vi "MotorNavigation.vi"() -> ()   [LabVIEW 2022 SP3]
panel:
  in  "Zero":bool
  in  "TZ [mm]":dbl format="%.3f"
  in  "TY [mm]":dbl format="%.3f"
  in  "TX [mm]":dbl format="%.3f"
  in  "SZ":u16(ring)=4000 items=["4000 ustep/s"=4000, "2000 ustep/s"=2000, "1000 ustep/s"=1000]
  in  "SY":u16(ring)=4000 items=["4000 ustep/s"=4000, "2000 ustep/s"=2000, "1000 ustep/s"=1000]
  in  "SX":u16(ring)=4000 items=["6000 ustep/s"=6000, "4000 ustep/s"=4000, "2000 ustep/s"=2000, "1000 ustep/s"=1000]
  out "Z [mm]":dbl format="%.3f"
  out "Y [mm]":dbl format="%.3f"
  out "X [mm]":dbl format="%.3f"
  in  "ustepZ":u16(ring)=4 items=["full"=1, "1/2"=2, "1/4"=4, "1/8"=8, "1/16"=16]
  in  "ustepY":u16(ring)=4 items=["full"=1, "1/2"=2, "1/4"=4, "1/8"=8, "1/16"=16]
  in  "ustepX":u16(ring)=4 items=["full"=1, "1/2"=2, "1/4"=4, "1/8"=8, "1/16"=16]
  in  "Abort":bool
  out "Moving":bool
  in  "Motor VISA":refnum<visa-resource-name>="COM4"
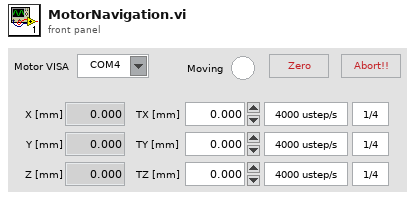
[diagram p1: front panel]
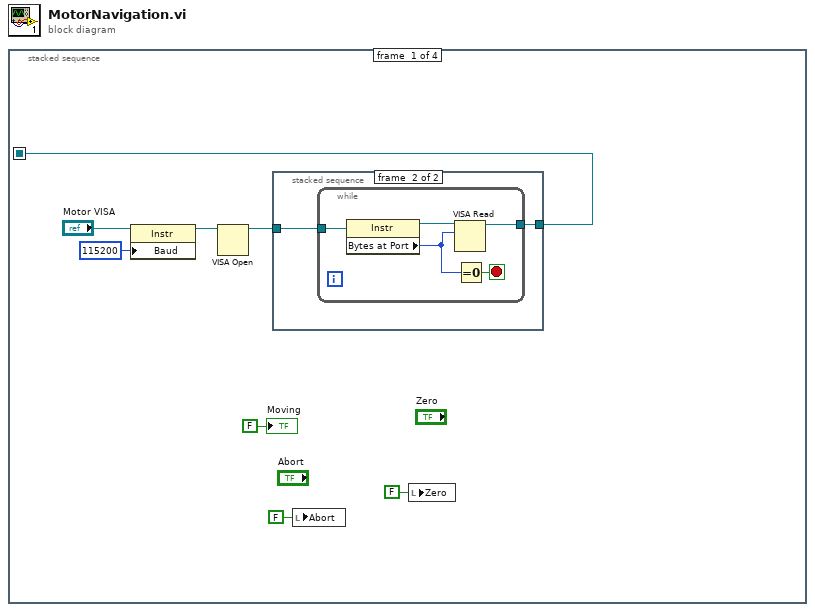
[diagram p0: block diagram]
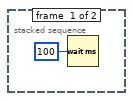
[diagram p2: hidden frame]
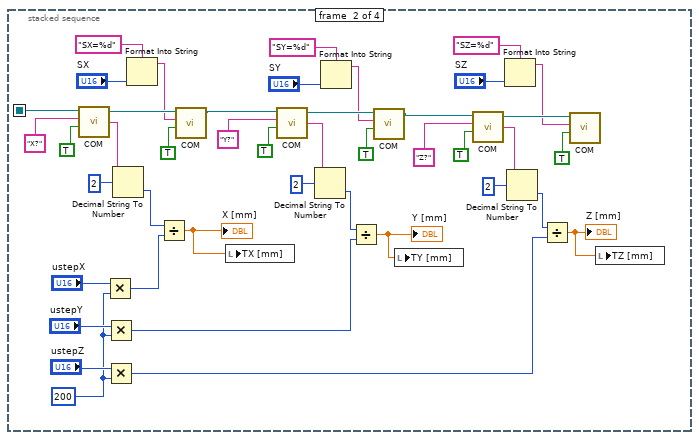
[diagram p3: hidden frame]
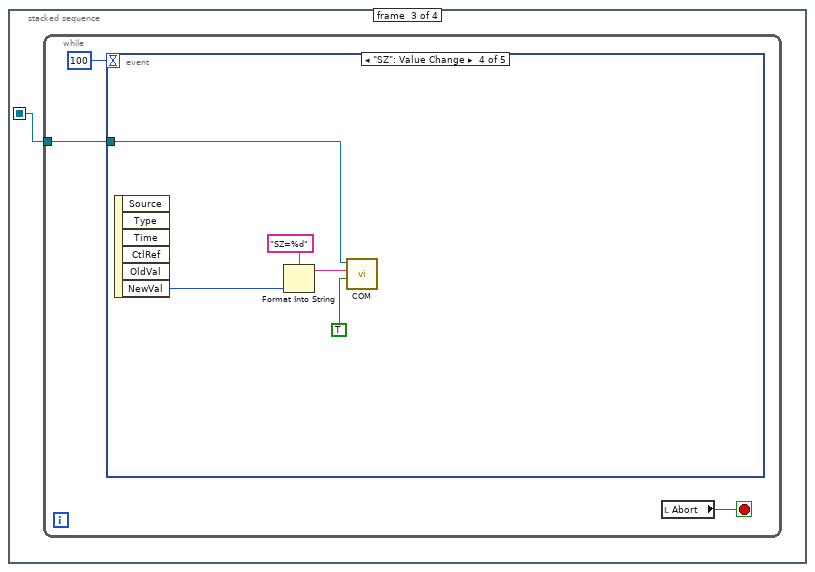
[diagram p4: hidden frame]
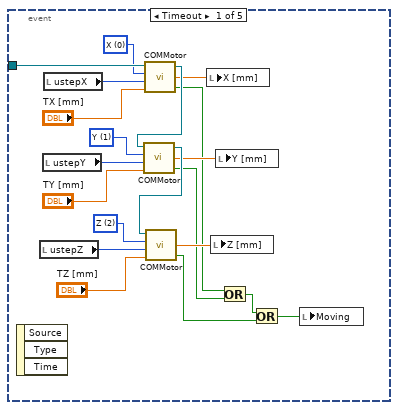
[diagram p5: hidden frame]
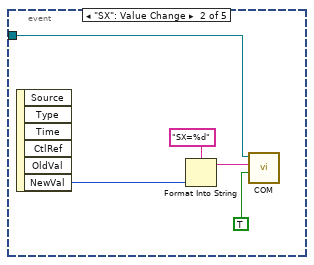
[diagram p6: hidden frame]
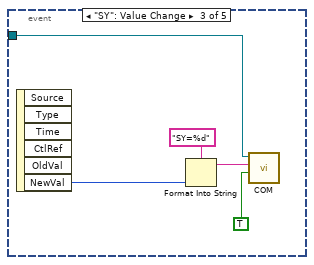
[diagram p7: hidden frame]
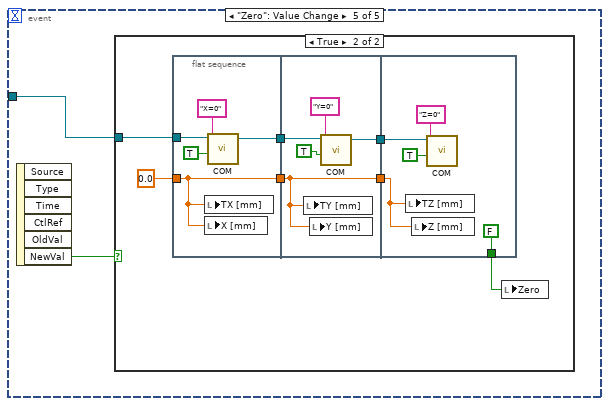
[diagram p8: hidden frame]
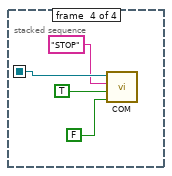
[diagram p10: hidden frame]
diagram:
  n1 = stacked-sequence {
    seq-local: [w4 _ _ _] -> [_ w59 w60 w126]
    frame #0 {
      n2 = property class="Instr"(reference="Motor VISA", "Baud"=u32 115200 ("Serial Settings:Baud Rate")) -> (reference out=w6:refnum<visa-resource-name>)  [unwired: 1 in, 1 out]
      n3 = VISA Open(VISA resource name=w6) -> (VISA resource name=w5:refnum<visa-resource-name>)  [unwired: 4 in, 1 out]
      n4 = stacked-sequence {
        tunnel: w5 -> [_ w11]
        tunnel: [_ w10] -> w4
        frame #0 {
          n5 = Wait (ms)(milliseconds to wait=u32 100) -> ()  [unwired: 1 out]
        }
        frame #1 {
          n6 = while {
            tunnel: w11 -> [w16]
            tunnel: [w12] -> w10
            stop <- w13 stop-if-true
            n7 = property class="Instr"(reference=w16) -> (reference out=w15:refnum<visa-resource-name>, "Bytes at Port"=w14:u32)  [unwired: 1 in, 1 out]
            n8 = VISA Read(VISA resource name=w15, byte count=w14) -> (VISA resource name out=w12:refnum<visa-resource-name>)  [unwired: 1 in, 3 out]
            n9 = Equal To 0?(x=w14) -> (x = 0?=w13:bool)
          }
        }
      }
      n10 = local write "Abort"(FALSE ("Abort")) -> ()
      n11 = local write "Zero"(FALSE ("Zero")) -> ()
      "Moving" <- FALSE ("Moving")
    }
    frame #1 {
      w39 = 200
      n12 = call "COM.vi"("Write?"=TRUE, "command"="X?", "VISA in"=w59) -> ("reply"=w44:string, "VISA out"=w55:refnum<visa-resource-name>)  [unwired: 1 in, 1 out]
      n13 = Multiply(x="ustepX", y=w39) -> (x*y=w37:i32)
      n14 = Multiply(x="ustepY", y=w39) -> (x*y=w31:i32)
      n15 = Multiply(x="ustepZ", y=w39) -> (x*y=w29:i32)
      n16 = Decimal String To Number(string=w44, offset=2 ("offset (0)")) -> (number=w38:i32)  [unwired: 1 in, 1 out]
      n17 = Format Into String(format string="SX=%d" ("command"), "SX") -> (resulting string=w26:string)  [unwired: 2 in, 1 out]
      n18 = Divide(x=w38, y=w37) -> (x/y=w19:dbl)
      "X [mm]" <- w19
      n19 = call "COM.vi"("Write?"=TRUE, "command"=w26, "VISA in"=w55) -> ("VISA out"=w46:refnum<visa-resource-name>)  [unwired: 1 in, 2 out]
      n20 = local write "TX [mm]"(w19) -> ()
      n21 = call "COM.vi"("Write?"=TRUE, "command"="Y?", "VISA in"=w46) -> ("reply"=w34:string, "VISA out"=w51:refnum<visa-resource-name>)  [unwired: 1 in, 1 out]
      n22 = Decimal String To Number(string=w34, offset=2 ("offset (0)")) -> (number=w32:i32)  [unwired: 1 in, 1 out]
      n23 = Format Into String(format string="SY=%d" ("command"), "SY") -> (resulting string=w21:string)  [unwired: 2 in, 1 out]
      n24 = Divide(x=w32, y=w31) -> (x/y=w17:dbl)
      "Y [mm]" <- w17
      n25 = call "COM.vi"("Write?"=TRUE, "command"=w21, "VISA in"=w51) -> ("VISA out"=w45:refnum<visa-resource-name>)  [unwired: 1 in, 2 out]
      n26 = local write "TY [mm]"(w17) -> ()
      n27 = call "COM.vi"("Write?"=TRUE, "command"="Z?", "VISA in"=w45) -> ("reply"=w33:string, "VISA out"=w47:refnum<visa-resource-name>)  [unwired: 1 in, 1 out]
      n28 = Format Into String(format string="SZ=%d" ("command"), "SZ") -> (resulting string=w20:string)  [unwired: 2 in, 1 out]
      n29 = Decimal String To Number(string=w33, offset=2 ("offset (0)")) -> (number=w30:i32)  [unwired: 1 in, 1 out]
      n30 = Divide(x=w30, y=w29) -> (x/y=w18:dbl)
      "Z [mm]" <- w18
      n31 = call "COM.vi"("Write?"=TRUE, "command"=w20, "VISA in"=w47) -> ()  [unwired: 1 in, 3 out]
      n32 = local write "TZ [mm]"(w18) -> ()
    }
    frame #2 {
      n33 = while {
        tunnel: w60 -> [w62]
        stop <- w61 stop-if-true
        n34 = event shown="[3] \"SZ\": Value Change" {
          selector: _ -> [_ _ _ _ _]
          dyn-events: _ -> [_ _ _ _ _]
          timeout: 100 -> [_ _ _ _ _]
          tunnel: w62 -> [w80 w85 w90 w95 w99]
          event Timeout {
            w73 = u16 2 items=["X", "Y", "Z"] ("axis")
            w77 = u16 1 items=["X", "Y", "Z"] ("axis")
            w79 = u16 0 items=["X", "Y", "Z"] ("axis")
            n35 = event-data() -> ()  [unwired: 1 in, 3 out]
            n36 = local read "ustepZ"() -> (w74:u16)
            n37 = local read "ustepY"() -> (w76:u16)
            n38 = local read "ustepX"() -> (w78:u16)
            n39 = call "COMMotor.vi"("Target [mm]"="TX [mm]", "ustep"=w78, "axis"=w79, "VISA in"=w80) -> ("Moving"=w66:bool, "Position [mm]"=w81:dbl, "VISA out"=w83:refnum<visa-resource-name>)
            n40 = call "COMMotor.vi"("Target [mm]"="TY [mm]", "ustep"=w76, "axis"=w77, "VISA in"=w83) -> ("Moving"=w65:bool, "Position [mm]"=w69:dbl, "VISA out"=w75:refnum<visa-resource-name>)
            n41 = call "COMMotor.vi"("Target [mm]"="TZ [mm]", "ustep"=w74, "axis"=w73, "VISA in"=w75) -> ("Moving"=w64:bool, "Position [mm]"=w68:dbl)  [unwired: 1 out]
            n42 = local write "X [mm]"(w81) -> ()
            n43 = local write "Z [mm]"(w68) -> ()
            n44 = local write "Y [mm]"(w69) -> ()
            n45 = Or(x=w66, y=w65) -> (x .or. y?=w67:bool)
            n46 = Or(x=w67, y=w64) -> (x .or. y?=w82:bool)
            n47 = local write "Moving"(w82) -> ()
          }
          event "SX": Value Change {
            n48 = event-data() -> ("NewVal"=w87:u16)  [unwired: 1 in, 5 out]
            n49 = Format Into String(format string="SX=%d" ("command"), w87) -> (resulting string=w86:string)  [unwired: 2 in, 1 out]
            n50 = call "COM.vi"("Write?"=TRUE, "command"=w86, "VISA in"=w85) -> ()  [unwired: 1 in, 3 out]
          }
          event "SY": Value Change {
            n51 = event-data() -> ("NewVal"=w92:u16)  [unwired: 1 in, 5 out]
            n52 = Format Into String(format string="SY=%d" ("command"), w92) -> (resulting string=w91:string)  [unwired: 2 in, 1 out]
            n53 = call "COM.vi"("Write?"=TRUE, "command"=w91, "VISA in"=w90) -> ()  [unwired: 1 in, 3 out]
          }
          event "SZ": Value Change {
            n54 = event-data() -> ("NewVal"=w97:u16)  [unwired: 1 in, 5 out]
            n55 = Format Into String(format string="SZ=%d" ("command"), w97) -> (resulting string=w96:string)  [unwired: 2 in, 1 out]
            n56 = call "COM.vi"("Write?"=TRUE, "command"=w96, "VISA in"=w95) -> ()  [unwired: 1 in, 3 out]
          }
          event "Zero": Value Change {
            n57 = event-data() -> ("NewVal"=w100:bool)  [unwired: 1 in, 5 out]
            n58 = case shown="True" w100 {
              tunnel: w99 -> [_ w107]
              frame False {
              }
              frame True {
                n59 = flat-sequence {
                  tunnel: w107 -> [w112]
                  tunnel: 0.0 ("TX [mm]") -> [w110]
                  tunnel: [w110] -> w105
                  tunnel: [w108] -> w103
                  tunnel: w105 -> [w117]
                  tunnel: [w117] -> w104
                  tunnel: w103 -> [w114]
                  tunnel: [w113] -> w102
                  tunnel: w104 -> [w122]
                  tunnel: w102 -> [w119]
                  tunnel: [FALSE ("Zero")] -> w101
                  frame #0 {
                    n60 = local write "TX [mm]"(w110) -> ()
                    n61 = local write "X [mm]"(w110) -> ()
                    n62 = call "COM.vi"("Write?"=TRUE, "command"="X=0", "VISA in"=w112) -> ("VISA out"=w108:refnum<visa-resource-name>)  [unwired: 1 in, 2 out]
                  }
                  frame #1 {
                    n63 = local write "TY [mm]"(w117) -> ()
                    n64 = local write "Y [mm]"(w117) -> ()
                    n65 = call "COM.vi"("Write?"=TRUE, "command"="Y=0", "VISA in"=w114) -> ("VISA out"=w113:refnum<visa-resource-name>)  [unwired: 1 in, 2 out]
                  }
                  frame #2 {
                    n66 = local write "TZ [mm]"(w122) -> ()
                    n67 = local write "Z [mm]"(w122) -> ()
                    n68 = call "COM.vi"("Write?"=TRUE, "command"="Z=0", "VISA in"=w119) -> ()  [unwired: 1 in, 3 out]
                  }
                }
                n69 = local write "Zero"(w101) -> ()
              }
            }
          }
        }
        n70 = local read "Abort"() -> (w61:bool)
      }
    }
    frame #3 {
      n71 = call "COM.vi"("Read?"=FALSE, "Write?"=TRUE, "command"="STOP", "VISA in"=w126) -> ()  [unwired: 3 out]
    }
  }
